vi "Configuration as JSON.vi"(8 "error in (no error)":errorcluster, 11 "Device in":refnum<class "Device.lvclass">) -> (0 "error out":errorcluster, 1 "JSON Data":string, 2 "Version":u32, 3 "Device out":refnum<class "Device.lvclass">)   [LabVIEW 2015, in "IBEX Device.lvlib" / "Device.lvclass"]
doc: "Provides a means of exporting the current Device configuration as JSON data."
uses:
  Device.lvclass
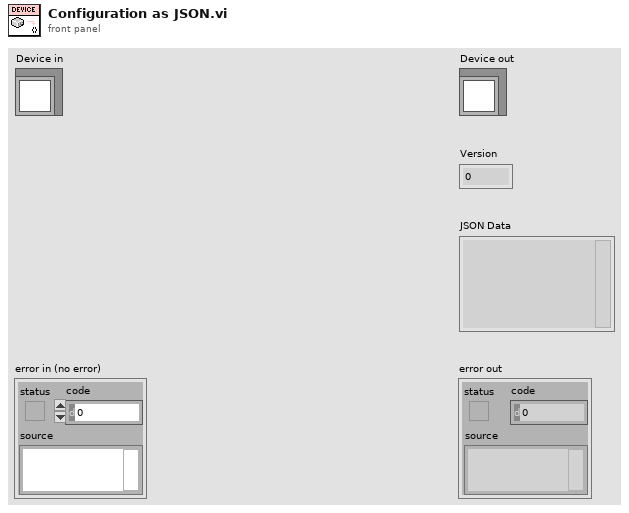
[diagram p1: front panel]
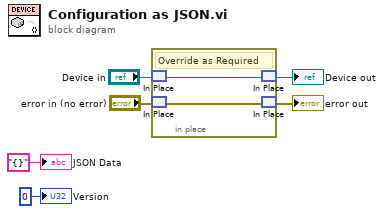
[diagram p0: block diagram]
diagram:
  n1 = in-place {
    # "Override as Required"
    n2 = in-place-match #1("Device in") -> (w8:refnum<class "Device.lvclass">)
    n3 = in-place-match #2("error in (no error)") -> (w7:errorcluster)
    n4 = in-place-match #1(w8) -> (→"Device out":refnum<class "Device.lvclass">)
    n5 = in-place-match #2(w7) -> (→"error out":errorcluster)
  }
  "JSON Data" <- "{}" ("JSON Data")
  "Version" <- u32 0 ("Version")
